vi "unpackPowerInfo.vi"(4 "长度":i32, 5 "数据":u8[](array[numeric]) format="%.0x") -> (1 "电能信息":T1)   [LabVIEW 2014]
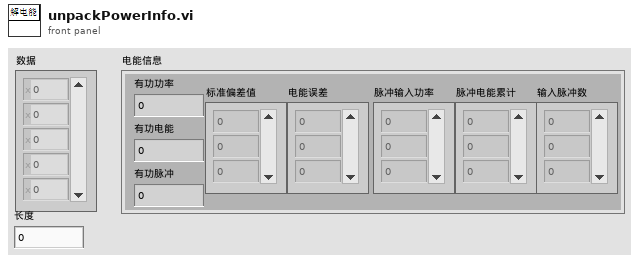
[diagram p1: front panel]
types:
  T1 = cluster{"有功功率":sgl, "有功电能":sgl, "有功脉冲":u64, "标准偏差值":sgl[], "电能误差":sgl[], "脉冲输入功率":sgl[], "脉冲电能累计":sgl[], "输入脉冲数":sgl[]}
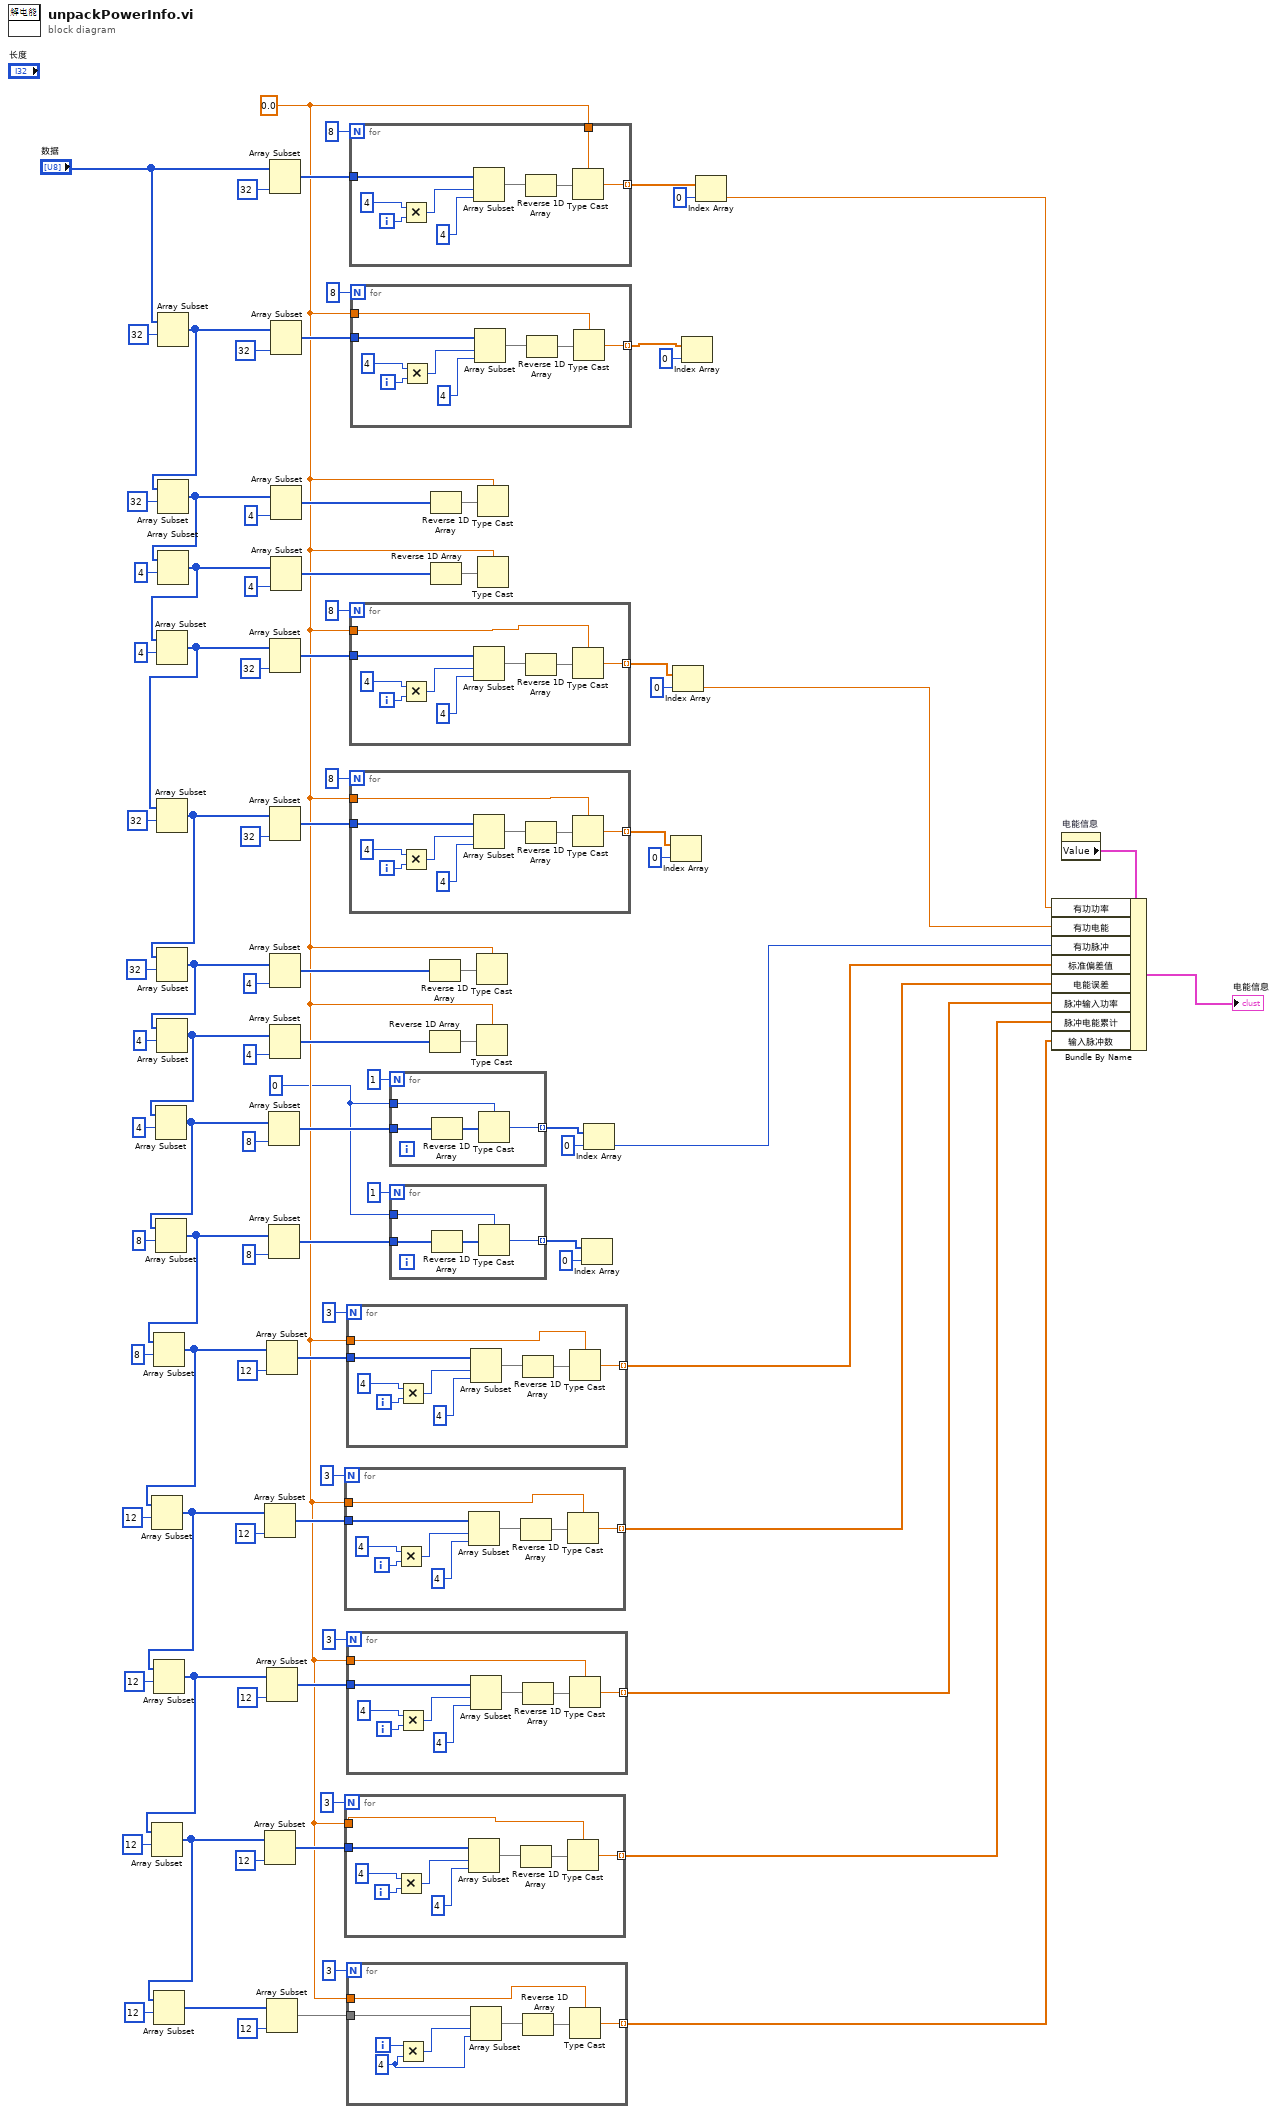
[diagram p0: block diagram]
diagram:
  w18 = u64 0
  w19 = sgl 0.0
  n1 = Array Subset(array="数据", index=32 ("索引")) -> (w91:u8[])  [unwired: 1 in]
  n2 = Array Subset(array=w91, index=32 ("索引")) -> (w82:u8[])  [unwired: 1 in]
  n3 = Array Subset(array=w82, index=4 ("索引")) -> (w77:u8[])  [unwired: 1 in]
  n4 = Array Subset(array=w77, index=4 ("索引")) -> (w72:u8[])  [unwired: 1 in]
  n5 = Array Subset(array=w72, index=32 ("索引")) -> (w62:u8[])  [unwired: 1 in]
  n6 = Array Subset(array=w62, index=32 ("索引")) -> (w71:u8[])  [unwired: 1 in]
  n7 = Array Subset(array=w71, index=4 ("索引")) -> (w58:u8[])  [unwired: 1 in]
  n8 = Array Subset(array=w58, index=4 ("索引")) -> (w54:u8[])  [unwired: 1 in]
  n9 = Array Subset(array=w54, index=8 ("索引")) -> (w49:u8[])  [unwired: 1 in]
  n10 = Array Subset(array=w49, index=8 ("索引")) -> (w44:u8[])  [unwired: 1 in]
  n11 = Array Subset(array=w44, index=12 ("索引")) -> (w34:u8[])  [unwired: 1 in]
  n12 = Array Subset(array=w34, index=12 ("索引")) -> (w43:u8[])  [unwired: 1 in]
  n13 = Array Subset(array=w43, index=12 ("索引")) -> (w29:u8[])  [unwired: 1 in]
  n14 = Array Subset(array=w29, index=12 ("索引")) -> (w20:u8[])  [unwired: 1 in]
  n15 = Array Subset(array=w34, length=12 ("长度")) -> (w47:u8[])  [unwired: 1 in]
  n16 = Array Subset(array=w29, length=12 ("长度")) -> (w40:u8[])  [unwired: 1 in]
  n17 = Array Subset(array=w44, length=12 ("长度")) -> (w51:u8[])  [unwired: 1 in]
  n18 = Array Subset(array=w43, length=12 ("长度")) -> (w37:u8[])  [unwired: 1 in]
  n19 = Array Subset(array=w20, length=12 ("长度")) -> (w32:u8[])  [unwired: 1 in]
  n20 = Array Subset(array=w54, length=8 ("长度")) -> (w61:u8[])  [unwired: 1 in]
  n21 = Array Subset(array=w49, length=8 ("长度")) -> (w55:u8[])  [unwired: 1 in]
  n22 = Array Subset(array="数据", length=32 ("长度")) -> (w97:u8[])  [unwired: 1 in]
  n23 = Array Subset(array=w72, length=32 ("长度")) -> (w79:u8[])  [unwired: 1 in]
  n24 = Array Subset(array=w62, length=32 ("长度")) -> (w75:u8[])  [unwired: 1 in]
  n25 = Array Subset(array=w71, length=4 ("长度")) -> (w66:u8[])  [unwired: 1 in]
  n26 = Array Subset(array=w58, length=4 ("长度")) -> (w67:u8[])  [unwired: 1 in]
  n27 = Array Subset(array=w91, length=32 ("长度")) -> (w94:u8[])  [unwired: 1 in]
  n28 = Array Subset(array=w82, length=4 ("长度")) -> (w87:u8[])  [unwired: 1 in]
  n29 = Array Subset(array=w77, length=4 ("长度")) -> (w86:u8[])  [unwired: 1 in]
  n30 = for {
    N: 3 -> [_]
    tunnel: w47 -> [w107]
    tunnel: [w100] -> w22 mode=indexing
    tunnel: w19 -> [w99]
    i -> [w103]
    n31 = Multiply(x=4, y=w103) -> (x*y=w105:i32)
    n32 = Array Subset(array=w107, index=w105, length=4 ("长度")) -> (w101:u8[])
    n33 = Reverse 1D Array(array=w101) -> (reversed array=w102:u8[])
    n34 = Type Cast(type=w99, x=w102) -> (*(type *) &x=w100:sgl)
  }
  n35 = for {
    N: 3 -> [_]
    tunnel: w40 -> [w116]
    tunnel: [w109] -> w24 mode=indexing
    tunnel: w19 -> [w108]
    i -> [w112]
    n36 = Multiply(x=4, y=w112) -> (x*y=w114:i32)
    n37 = Array Subset(array=w116, index=w114, length=4 ("长度")) -> (w110:u8[])
    n38 = Reverse 1D Array(array=w110) -> (reversed array=w111:u8[])
    n39 = Type Cast(type=w108, x=w111) -> (*(type *) &x=w109:sgl)
  }
  n40 = for {
    N: 3 -> [_]
    tunnel: w51 -> [w125]
    tunnel: [w118] -> w21 mode=indexing
    tunnel: w19 -> [w117]
    i -> [w121]
    n41 = Multiply(x=4, y=w121) -> (x*y=w123:i32)
    n42 = Array Subset(array=w125, index=w123, length=4 ("长度")) -> (w119:u8[])
    n43 = Reverse 1D Array(array=w119) -> (reversed array=w120:u8[])
    n44 = Type Cast(type=w117, x=w120) -> (*(type *) &x=w118:sgl)
  }
  n45 = for {
    N: 3 -> [_]
    tunnel: w37 -> [w134]
    tunnel: [w127] -> w23 mode=indexing
    tunnel: w19 -> [w126]
    i -> [w130]
    n46 = Multiply(x=4, y=w130) -> (x*y=w132:i32)
    n47 = Array Subset(array=w134, index=w132, length=4 ("长度")) -> (w128:u8[])
    n48 = Reverse 1D Array(array=w128) -> (reversed array=w129:u8[])
    n49 = Type Cast(type=w126, x=w129) -> (*(type *) &x=w127:sgl)
  }
  n50 = for {
    N: 3 -> [_]
    tunnel: w32 -> [w142]
    tunnel: [w138] -> w25 mode=indexing
    tunnel: w19 -> [w135]
    i -> [w137]
    w136 = 4 ("长度")
    n51 = Multiply(x=w137, y=w136) -> (x*y=w141:i32)
    n52 = Array Subset(array=w142, index=w141, length=w136) -> (w139:u8[])
    n53 = Reverse 1D Array(array=w139) -> (reversed array=w140:u8[])
    n54 = Type Cast(type=w135, x=w140) -> (*(type *) &x=w138:sgl)
  }
  n55 = for {
    N: 8 -> [_]
    tunnel: w97 -> [w151]
    tunnel: [w144] -> w15 mode=indexing
    tunnel: w19 -> [w143]
    i -> [w147]
    n56 = Multiply(x=4, y=w147) -> (x*y=w149:i32)
    n57 = Array Subset(array=w151, index=w149, length=4 ("长度")) -> (w145:u8[])
    n58 = Reverse 1D Array(array=w145) -> (reversed array=w146:u8[])
    n59 = Type Cast(type=w143, x=w146) -> (*(type *) &x=w144:sgl)
  }
  n60 = for {
    N: 8 -> [_]
    tunnel: w79 -> [w160]
    tunnel: [w153] -> w10 mode=indexing
    tunnel: w19 -> [w152]
    i -> [w156]
    n61 = Multiply(x=4, y=w156) -> (x*y=w158:i32)
    n62 = Array Subset(array=w160, index=w158, length=4 ("长度")) -> (w154:u8[])
    n63 = Reverse 1D Array(array=w154) -> (reversed array=w155:u8[])
    n64 = Type Cast(type=w152, x=w155) -> (*(type *) &x=w153:sgl)
  }
  n65 = for {
    N: 8 -> [_]
    tunnel: w75 -> [w169]
    tunnel: [w162] -> w8 mode=indexing
    tunnel: w19 -> [w161]
    i -> [w165]
    n66 = Multiply(x=4, y=w165) -> (x*y=w167:i32)
    n67 = Array Subset(array=w169, index=w167, length=4 ("长度")) -> (w163:u8[])
    n68 = Reverse 1D Array(array=w163) -> (reversed array=w164:u8[])
    n69 = Type Cast(type=w161, x=w164) -> (*(type *) &x=w162:sgl)
  }
  n70 = for {
    N: 8 -> [_]
    tunnel: w94 -> [w178]
    tunnel: [w171] -> w12 mode=indexing
    tunnel: w19 -> [w170]
    i -> [w174]
    n71 = Multiply(x=4, y=w174) -> (x*y=w176:i32)
    n72 = Array Subset(array=w178, index=w176, length=4 ("长度")) -> (w172:u8[])
    n73 = Reverse 1D Array(array=w172) -> (reversed array=w173:u8[])
    n74 = Type Cast(type=w170, x=w173) -> (*(type *) &x=w171:sgl)
  }
  n75 = for {
    N: 1 -> [_]
    tunnel: w61 -> [w182]
    tunnel: [w180] -> w5 mode=indexing
    tunnel: w18 -> [w179]
    n76 = Reverse 1D Array(array=w182) -> (reversed array=w181:u8[])
    n77 = Type Cast(type=w179, x=w181) -> (*(type *) &x=w180:u64)
  }
  n78 = for {
    N: 1 -> [_]
    tunnel: w55 -> [w186]
    tunnel: [w184] -> w4 mode=indexing
    tunnel: w18 -> [w183]
    n79 = Reverse 1D Array(array=w186) -> (reversed array=w185:u8[])
    n80 = Type Cast(type=w183, x=w185) -> (*(type *) &x=w184:u64)
  }
  n81 = Reverse 1D Array(array=w66) -> (reversed array=w65:u8[])
  n82 = Reverse 1D Array(array=w67) -> (reversed array=w68:u8[])
  n83 = Reverse 1D Array(array=w87) -> (reversed array=w88:u8[])
  n84 = Reverse 1D Array(array=w86) -> (reversed array=w85:u8[])
  n85 = Type Cast(type=w19, x=w65) -> ()  [unwired: 1 out]
  n86 = Type Cast(type=w19, x=w68) -> ()  [unwired: 1 out]
  n87 = Type Cast(type=w19, x=w88) -> ()  [unwired: 1 out]
  n88 = Type Cast(type=w19, x=w85) -> ()  [unwired: 1 out]
  n89 = Index Array(array=w4, index=0 ("索引")) -> ()  [unwired: 1 out]
  n90 = Index Array(array=w5, index=0 ("索引")) -> (element=w1:u64)
  n91 = Index Array(array=w8, index=0 ("索引")) -> ()  [unwired: 1 out]
  n92 = Index Array(array=w10, index=0 ("索引")) -> (element=w2:sgl)
  n93 = Index Array(array=w12, index=0 ("索引")) -> ()  [unwired: 1 out]
  n94 = Index Array(array=w15, index=0 ("索引")) -> (element=w3:sgl)
  n95 = property on="电能信息" class="Clust (严格)"() -> ("Value"=w26:T1)  [unwired: 2 in, 2 out]
  n96 = Bundle By Name(cluster=w26, "有功功率"=w3, "有功电能"=w2, "有功脉冲"=w1, "标准偏差值"=w21, "电能误差"=w22, "脉冲输入功率"=w23, "脉冲电能累计"=w24, "输入脉冲数"=w25) -> (→"电能信息":T1)
